vi "Main.vi"(10 "Sub Panel":refnum<vi>, 11 "Module Admin":refnum<class "Delacor_lib_QMH_Module Admin.lvclass">) -> ()   [LabVIEW 2020, in "Message Pane.lvlib"]
doc: "This template is based off of the Queued Message Handler design pattern and the Queued Message Handler project template that ships with LabVIEW.\n\nThe main difference is that the queue is private to this module and communication between modules is performed via Broadcast and Request events.\n\nRequest events are wrapped in public API methods and are handled in the Event Handling Loop (EHL) of this VI. Any module can register for Broadcast events sent by this module. The EHL generates messages based on user interface actions.\n\nThe Message Handling Loop (MHL) processes messages generated by the EHL, or by other messages. The messages are string values, so new messages can be added easily to the Message Cases case structure in the MHL. Each message cluster can also provide an optional value for Message Data, which is a variant that can be converted to whatever message-specific data is required.\n_____\nBased on Delacor QMH Project Template 5.0.0.82."
uses:
  Message Pane.lvlib
  <vilib>/Delacor/Delacor QMH/Libraries/Module Admin_class/Delacor_lib_QMH_Module Admin.lvclass
  Module Data--cluster.ctl
  Stop Argument--cluster.ctl
  <vilib>/Delacor/Delacor QMH/Libraries/Message Queue_class/Delacor_lib_QMH_Message Queue.lvclass/Delacor_lib_QMH_Message Queue.ctl
  <vilib>/Delacor/Delacor QMH/Libraries/Module Admin_class/Delacor_lib_QMH_Module Admin.lvclass/Delacor_lib_QMH_Module Admin.ctl
  Credit Update Argument--cluster.ctl
  Purchase action Argument--cluster.ctl
  SQLITE Inventory/Invetory Data Type.ctl
  <vilib>/Utility/miscctls.llb/LVPointTypeDef.ctl
  <vilib>/Delacor/Delacor QMH/Libraries/Message Queue_class/Delacor_lib_QMH_Enqueue Message (Single).vi
  <vilib>/Delacor/Delacor QMH/Libraries/Module Admin_class/Delacor_lib_QMH_Get External Launch.vi
  <vilib>/Utility/error.llb/Error Cluster From Error Code.vi
  <vilib>/ErrorRing/Error Ring.xnode
  <vilib>/Delacor/Delacor QMH/Libraries/Message Queue_class/Delacor_lib_QMH_Message Queue.lvclass
  SQLITE Inventory/SQLITE Inventory.lvlib
  Product Selecting Pane/Product Selecting Pane.lvlib
panel:
  out "Change":dbl
  out "Status":string
  out "Selected Product":string
  out "Credit":dbl
  out "error out":errorcluster
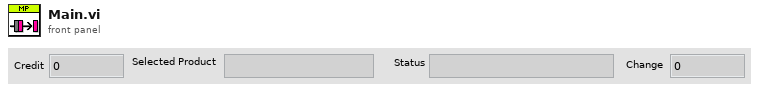
[diagram p1: front panel]
types:
  T1 = typedef "Message Pane.lvlib/Request Events--cluster.ctl" = cluster{"Stop Module":refnum<user-event>, "Show Panel":refnum<user-event>, "Hide Panel":refnum<user-event>, "Get Module Execution Status":refnum<user-event>, "Show Diagram":refnum<user-event>, "Credit Update":refnum<user-event>, "Purchase action":refnum<user-event>}
  T2 = typedef "Message Pane.lvlib/Module Data--cluster.ctl" = cluster{"Credit":dbl, "Status":string, "Change":dbl, "Product":string}
  T3 = enum32{"invalid lock state", "Not Locked", "Locked (No Password)", "Password-protected"}
  T4 = typedef "Message Pane.lvlib/Stop Argument--cluster.ctl" = cluster{"Origin":string, "Exit via Stop Module Req?":bool, "Wait for Module to stop?":bool}
  T5 = typedef "Message Pane.lvlib/Credit Update Argument--cluster.ctl" = cluster{"Numeric":dbl}
  T6 = typedef "Message Pane.lvlib/Purchase action Argument--cluster.ctl" = cluster{"Cluster":T7}
  T7 = typedef "Invetory Data Type.ctl" = cluster{"Name":string, "Price":dbl, "Stock":dbl}
  T8 = typedef "LVPointTypeDef.ctl" = cluster{"Horizontal":i16, "Vertical":i16}
  T9 = enum32{"Invalid", "Standard", "Closed", "Hidden", "Minimized", "Maximized"}
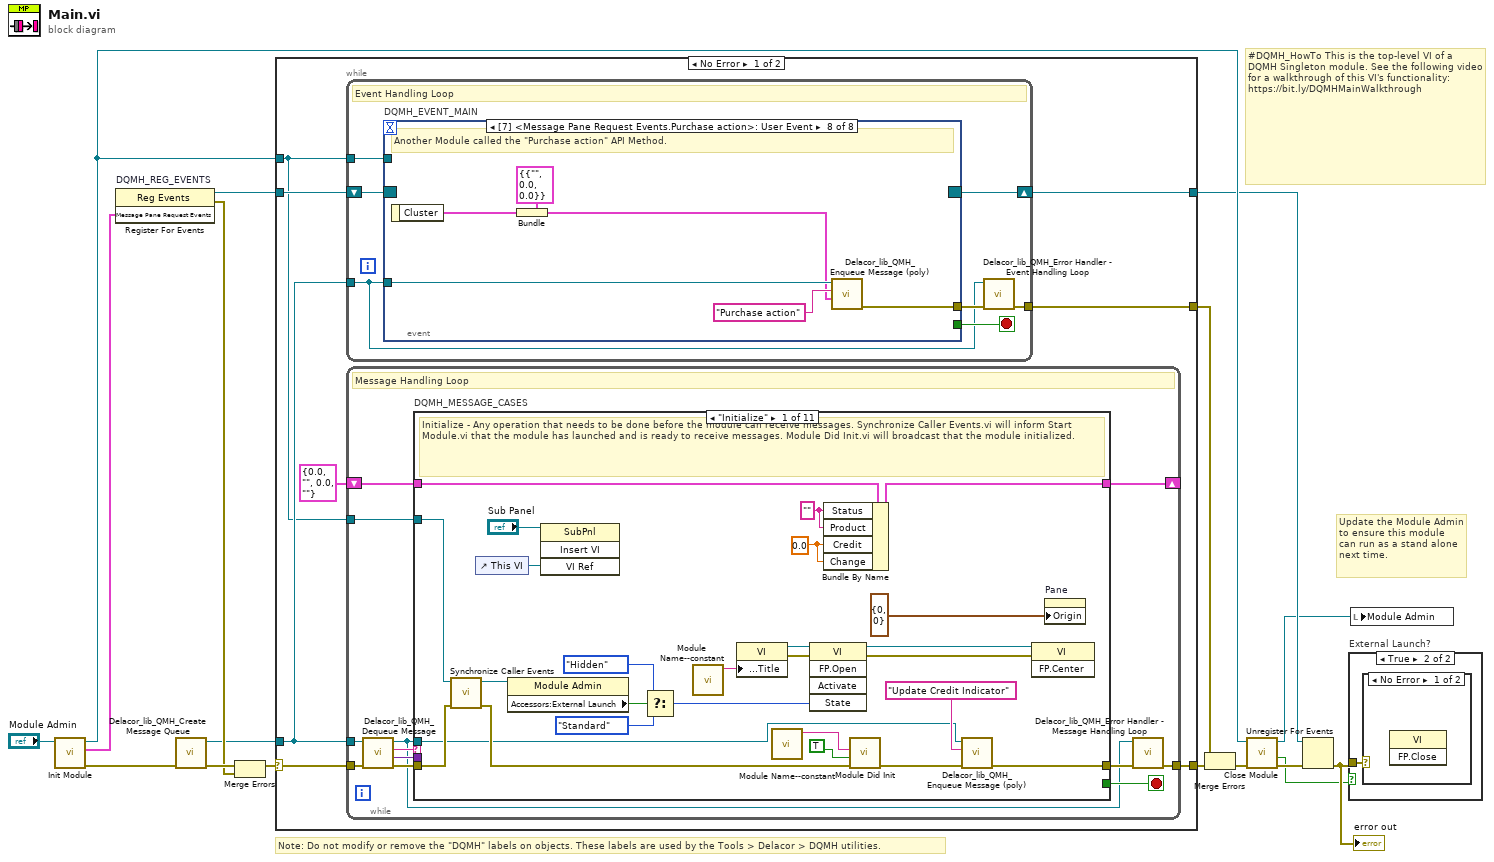
[diagram p0: block diagram]
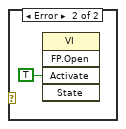
[diagram p3: hidden frame]
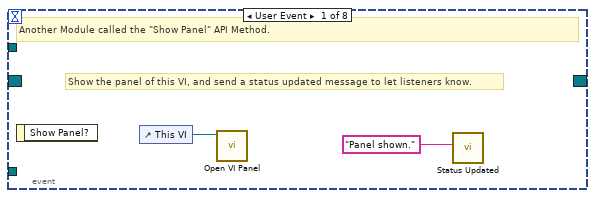
[diagram p4: hidden frame]
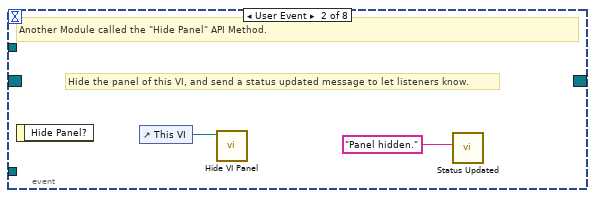
[diagram p5: hidden frame]
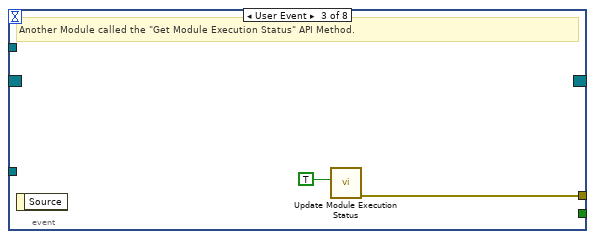
[diagram p6: hidden frame]
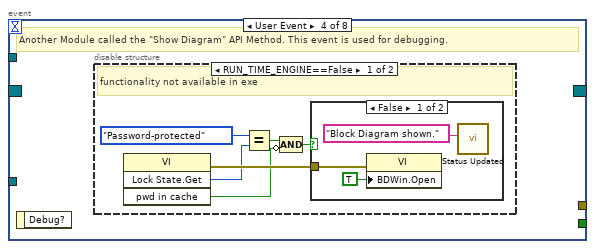
[diagram p7: hidden frame]
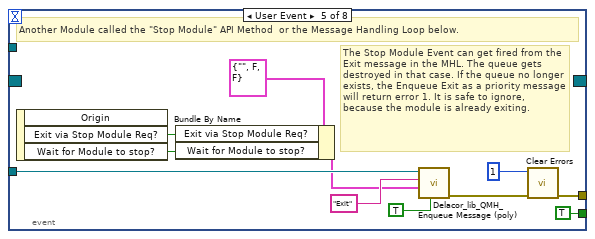
[diagram p10: hidden frame]
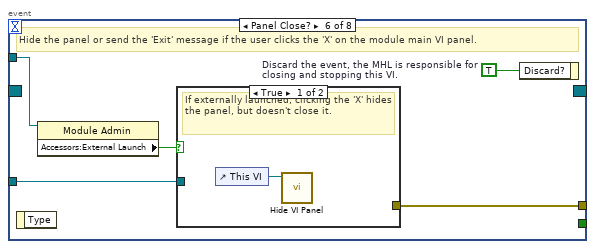
[diagram p11: hidden frame]
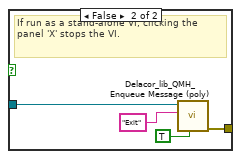
[diagram p12: hidden frame]
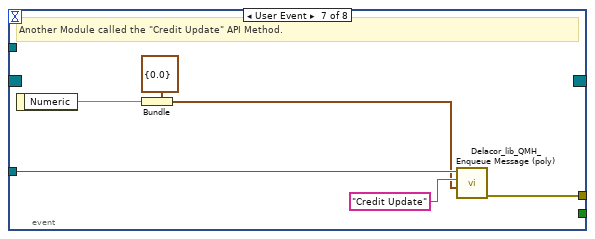
[diagram p13: hidden frame]
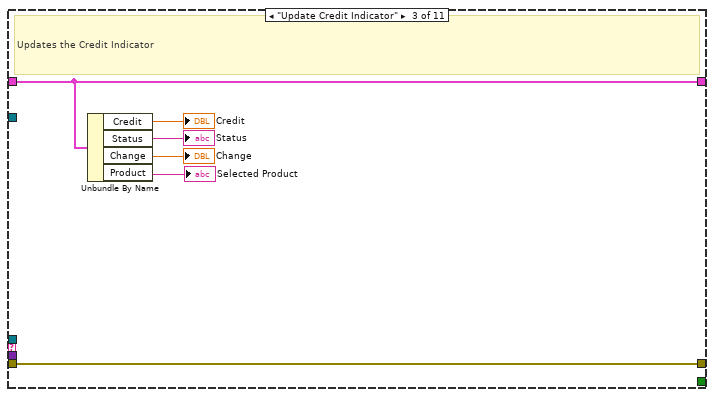
[diagram p15: hidden frame]
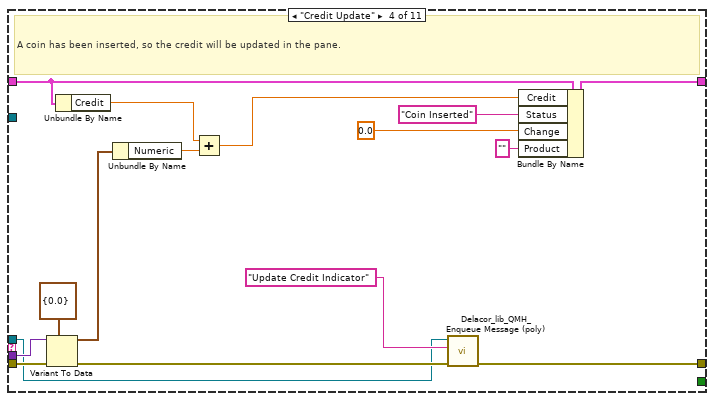
[diagram p16: hidden frame]
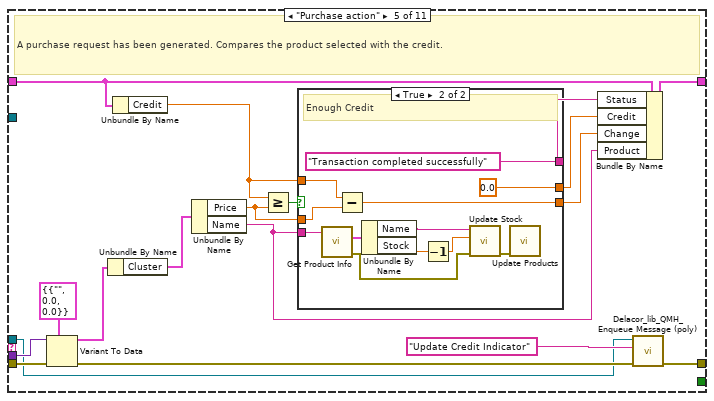
[diagram p17: hidden frame]
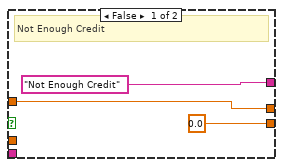
[diagram p18: hidden frame]
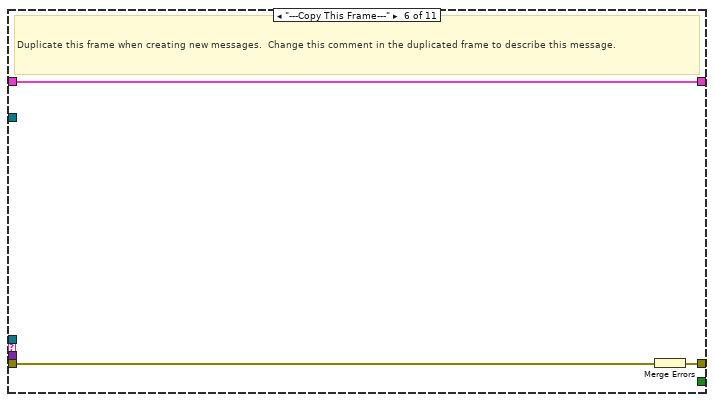
[diagram p19: hidden frame]
diagram:
  # "#DQMH_HowTo This is the top-level VI of a DQMH Singleton module. See the following video for a walkthrough of this VI's functionality: https://bit.ly/DQMHMainWalkthrough"
  # "Note: Do not modify or remove the \"DQMH\" labels on objects. These labels are used by the Tools > Delacor > DQMH utilities."
  # "Update the Module Admin to ensure this module can run as a stand alone next time."
  n1 = call "Init Module.vi"("Singleton Module Admin in"="Module Admin") -> ("error out"=w16:errorcluster, "Message Pane Request Events"=w5:T1, "Singleton Module Admin out"=w8:refnum<class "Delacor_lib_QMH_Module Admin.lvclass">)  [unwired: 8 in]
  n2 = register-events "DQMH_REG_EVENTS"(w5) -> (reference out=w6:refnum<event-registration>, error out=w9:errorcluster)  [unwired: 2 in]
  n3 = call <vilib>:"Delacor_lib_QMH_Create Message Queue.vi"("error in (no error)"=w16) -> ("error out"=w11:errorcluster, "Message Queue"=w4:refnum<class "Delacor_lib_QMH_Message Queue.lvclass">)  [unwired: 9 in]
  n4 = Merge Errors(w11, w9) -> (w10:errorcluster)
  n5 = case shown="No Error" w10 {
    selector: w10 -> [w23 w241]
    tunnel: [w25 w240] -> w17
    tunnel: [w22 w246] -> w7
    tunnel: w6 -> [w20 w246]
    tunnel: w4 -> [w19 w239]
    tunnel: [w24 _] -> w14
    tunnel: w8 -> [w18 w242]
    frame No Error {
      n6 = while {
        tunnel: w19 -> [w26]
        shift-right: [w29] -> w22
        shift-left: w20 -> [w30]
        tunnel: [w31] -> w24
        tunnel: w18 -> [w27]
        stop <- w28 stop-if-true
        # "Event Handling Loop"
        n7 = event "DQMH_EVENT_MAIN" shown="[7] <Message Pane Request Events.Purchase action>: User Event" {
          selector: w30 -> [_ _ _ _ _ _ _ _]
          dyn-events: [_ _ _ _ _ _ _ _] -> w29
          timeout: _ -> [_ _ _ _ _ _ _ _]
          tunnel: [_ _ _ _ TRUE ("Discard?") _ _ _] -> w28
          tunnel: w26 -> [_ _ _ _ w54 w61 w74 w80]
          tunnel: [_ _ w38 _ w57 w63 w69 w75] -> w32
          tunnel: w27 -> [_ _ _ _ _ w60 _ _]
          event User Event {
            # "Show the panel of this VI, and send a status updated message to let listeners know."
            # "Another Module called the \"Show Panel\" API Method."
            n8 = event-data() -> ()  [unwired: 1 in, 1 out]
            n9 = control-ref of="This VI"() -> (w34:refnum<vi>)
            n10 = call "Open VI Panel.vi"("VI"=w34) -> ()  [unwired: 10 in, 1 out]
            n11 = call "Status Updated.vi"("Status"="Panel shown." ("format string")) -> ()  [unwired: 10 in, 1 out]
          }
          event User Event {
            # "Hide the panel of this VI, and send a status updated message to let listeners know."
            # "Another Module called the \"Hide Panel\" API Method."
            n12 = event-data() -> ()  [unwired: 1 in, 1 out]
            n13 = control-ref of="This VI"() -> (w36:refnum<vi>)
            n14 = call "Hide VI Panel.vi"("VI"=w36) -> ()  [unwired: 10 in, 1 out]
            n15 = call "Status Updated.vi"("Status"="Panel hidden." ("format string")) -> ()  [unwired: 10 in, 1 out]
          }
          event User Event {
            # "Another Module called the \"Get Module Execution Status\" API Method."
            n16 = event-data() -> ()  [unwired: 1 in, 1 out]
            n17 = call "Update Module Execution Status.vi"("Running?"=TRUE) -> ("error out"=w38:errorcluster)  [unwired: 10 in]
          }
          event User Event {
            # "Another Module called the \"Show Diagram\" API Method. This event is used for debugging."
            n18 = event-data() -> ()  [unwired: 1 in, 1 out]
            n19 = disable-structure shown="RUN_TIME_ENGINE==False" {
              frame condition #0 (active) {
                # "functionality not available in exe"
                n20 = invoke class="VI" method="Lock State.Get"() -> (error out=w44:errorcluster, "Get Lock State"=w43:T3, "pwd in cache"=w40:bool)  [unwired: 4 in, 1 out]
                n21 = Equal?(x=T3."Password-protected", y=w43) -> (x = y?=w41:bool)
                n22 = Compound Arithmetic op=AND(w41, invert w40) -> (w39:bool)
                n23 = case shown="False" w39 {
                  tunnel: w44 -> [w47 _]
                  frame False {
                    n24 = property class="VI"(error in=w47, "BDWin.Open"=TRUE ("Block Diagram Window:Open")) -> ()  [unwired: 1 in, 2 out]
                    n25 = call "Status Updated.vi"("Status"="Block Diagram shown." ("format string")) -> ()  [unwired: 10 in, 1 out]
                  }
                  frame True {
                    # "Password-protected VI, and the password is not in the cache. Do not show the diagram."
                  }
                }
              }
              frame condition #1 {
              }
            }
          }
          event User Event {
            # "The Stop Module Event can get fired from the Exit message in the MHL. The queue gets destroyed in that case. If the queue no longer exists, the Enqueue Exit as a priority message will return error 1. It is safe to ignore, because the module is already exiting."
            # "Another Module called the \"Stop Module\" API Method  or the Message Handling Loop below."
            n26 = event-data() -> ("Exit via Stop Module Req?"=w50:bool, "Wait for Module to stop?"=w49:bool)  [unwired: 1 in, 1 out]
            n27 = Bundle By Name(cluster=T4 {"Origin"="", "Exit via Stop Module Req?"=FALSE, "Wait for Module to stop?"=FALSE} ("Stop Argument"), "Exit via Stop Module Req?"=w50, "Wait for Module to stop?"=w49) -> (w48:T4)
            n28 = call-poly <vilib>:"Delacor_lib_QMH_Enqueue Message (poly).vi"("Priority Message? (F)"=TRUE, "Message Data"=w48, "Message"="Exit", "Message Queue in"=w54) -> ("error out"=w58:errorcluster)  [unwired: 6 in, 1 out]
            n29 = call <vilib>:"Clear Errors.vi"("error in (no error)"=w58, "specific error code to clear (0: all)"=1) -> ("error out"=w57:errorcluster)  [unwired: 4 in, 1 out]
          }
          event Panel Close? {
            w62 = TRUE  # Discard the event, the MHL is responsible for closing and stopping this VI.
            # "Hide the panel or send the 'Exit' message if the user clicks the 'X' on the module main VI panel."
            n30 = event-data() -> ()  [unwired: 1 in, 1 out]
            n31 = property class="Module Admin"(reference=w60) -> ("Accessors:External Launch"=w59:bool)  [unwired: 1 in, 2 out]
            n32 = case shown="True" w59 {
              tunnel: w61 -> [_ w67]
              tunnel: [_ w68] -> w63
              frame True {
                # "If externally launched, clicking the 'X' hides the panel, but doesn't close it."
                n33 = control-ref of="This VI"() -> (w64:refnum<vi>)
                n34 = call "Hide VI Panel.vi"("VI"=w64) -> ()  [unwired: 10 in, 1 out]
              }
              frame False {
                # "If run as a stand-alone VI, clicking the panel 'X' stops the VI."
                n35 = call-poly <vilib>:"Delacor_lib_QMH_Enqueue Message (poly).vi"("Priority Message? (F)"=TRUE, "Message"="Exit", "Message Queue in"=w67) -> ("error out"=w68:errorcluster)  [unwired: 7 in, 1 out]
              }
            }
            n36 = event-data("Discard?"=w62) -> ()  [unwired: 1 in, 1 out]
          }
          event User Event {
            # "Another Module called the \"Credit Update\" API Method."
            n37 = event-data() -> ("Numeric"=w70:dbl)  [unwired: 1 in]
            n38 = Bundle(cluster=T5 {"Numeric"=0.0} ("Credit Update Argument"), "Numeric"=w70) -> (w71:T5)
            n39 = call-poly <vilib>:"Delacor_lib_QMH_Enqueue Message (poly).vi"("Message Data"=w71, "Message"="Credit Update", "Message Queue in"=w74) -> ("error out"=w69:errorcluster)  [unwired: 7 in, 1 out]
          }
          event User Event {
            # "Another Module called the \"Purchase action\" API Method."
            n40 = event-data() -> ("Cluster"=w76:T7)  [unwired: 1 in]
            n41 = Bundle(cluster=T6 {"Cluster"={"Name"="", "Price"=0.0, "Stock"=0.0}} ("Purchase action Argument"), "Cluster"=w76) -> (w77:T6)
            n42 = call-poly <vilib>:"Delacor_lib_QMH_Enqueue Message (poly).vi"("Message Data"=w77, "Message"="Purchase action", "Message Queue in"=w80) -> ("error out"=w75:errorcluster)  [unwired: 7 in, 1 out]
          }
        }
        n43 = call-dynamic "Delacor_lib_QMH_Error Handler - Event Handling Loop.vi"("error in (no error)"=w32, "Message Queue in"=w26) -> ("dup error in"=w31:errorcluster)  [unwired: 8 in, 1 out]
      }
      n44 = while {
        tunnel: w19 -> [w83]
        shift-right: [w87] -> _
        shift-left: T2 {"Credit"=0.0, "Status"="", "Change"=0.0, "Product"=""} ("Data Cluster") -> [w88]
        tunnel: w23 -> [w91]
        tunnel: [w89] -> w25
        tunnel: w18 -> [w81]
        stop <- w86 stop-if-true
        # "Message Handling Loop"
        n45 = call-dynamic "Delacor_lib_QMH_Dequeue Message.vi"("error in (no error)"=w91, "Message Queue in"=w83) -> ("error out"=w90:errorcluster, "Message Data"=w84:variant, "Message"=w85:string, "Message Queue out"=w82:refnum<class "Delacor_lib_QMH_Message Queue.lvclass">)  [unwired: 6 in]
        n46 = case "DQMH_MESSAGE_CASES" shown="\"Initialize\"" w85 {
          selector: w85 -> [_ _ _ _ _ _ _ _ _ _ w226]
          tunnel: w82 -> [w95 _ _ w130 w145 _ _ _ w196 w218 _]
          tunnel: w90 -> [w116 w120 w126 w142 w160 w178 w180 w185 w203 w224 w228]
          tunnel: [w97 w120 w126 w133 w146 w177 w180 w184 w199 w221 w229] -> w92
          tunnel: w88 -> [w106 w119 w125 w137 w156 w176 w179 w182 w198 w217 w227]
          tunnel: [w105 w119 w125 w138 w154 w176 w179 w182 w198 w217 w227] -> w87
          tunnel: [_ _ _ _ _ _ _ _ _ w216 _] -> w86
          tunnel: w84 -> [_ _ _ w141 w159 _ _ _ w197 w215 _]
          tunnel: w81 -> [w107 _ _ _ _ _ _ _ w195 w210 _]
          frame "Initialize" {
            w99 = 0.0
            w100 = "" ("Status")
            # "Initialize - Any operation that needs to be done before the module can receive messages. Synchronize Caller Events.vi will inform Start Module.vi that the module has launched and is ready to receive messages. Module Did Init.vi will broadcast that the module initialized."
            n47 = call "Synchronize Caller Events.vi"("error in (no error)"=w116, "Singleton Module Admin in"=w107) -> ("error out"=w115:errorcluster, "Singleton Module Admin out"=w102:refnum<class "Delacor_lib_QMH_Module Admin.lvclass">)  [unwired: 8 in]
            n48 = control-ref of="This VI"() -> (w93:refnum<vi>)
            n49 = property class="Module Admin"(reference=w102) -> ("Accessors:External Launch"=w111:bool)  [unwired: 1 in, 2 out]
            n50 = invoke class="SubPnl" method="Insert VI"(reference="Sub Panel", "VI Ref"=w93) -> ()  [unwired: 2 in, 4 out]
            n51 = Select(t=T9."Hidden" ("State"), s=w111, f=T9."Standard" ("State")) -> (s? t:f=w108:T9)
            n52 = call "Module Name--constant.vi"() -> ("Module Name"=w114:string)  [unwired: 11 in]
            n53 = property class="VI"("Front Panel.Title"=w114) -> (reference out=w113:refnum<vi>, error out=w118:errorcluster)  [unwired: 2 in]
            n54 = call "Module Name--constant.vi"() -> ("Module Name"=w103:string)  [unwired: 11 in]
            n55 = invoke class="VI" method="FP.Open"(reference=w113, error in=w118, "State"=w108) -> (reference out=w112:refnum<vi>, error out=w117:errorcluster)  [unwired: 2 in, 3 out]
            n56 = Bundle By Name(cluster=w106, "Status"=w100, "Product"=w100, "Credit"=w99, "Change"=w99) -> (w105:T2)
            n57 = call "Module Did Init.vi"("error in (no error)"=w115, "Initialized?"=TRUE, "Origin"=w103) -> ("error out"=w98:errorcluster)  [unwired: 8 in]
            n58 = call-poly <vilib>:"Delacor_lib_QMH_Enqueue Message (poly).vi"("error in (no error)"=w98, "Message"="Update Credit Indicator", "Message Queue in"=w95) -> ("error out"=w97:errorcluster)  [unwired: 7 in, 1 out]
            n59 = invoke class="VI" method="FP.Center"(reference=w112, error in=w117) -> ()  [unwired: 1 in, 3 out]
            n60 = property on="Pane" class="Pane"("Origin"=T8 {"Horizontal"=0, "Vertical"=0}) -> ()  [unwired: 2 in, 2 out]
          }
          frame "--- Module Specific ---" {
            # "Separator -- The following cases handle messages specific to this Module."
          }
          frame "Update Credit Indicator" {
            # "Updates the Credit Indicator"
            n61 = Unbundle By Name(w125) -> ("Credit"=→"Credit":dbl, "Status"=→"Status":string, "Change"=→"Change":dbl, "Product"=→"Selected Product":string)
          }
          frame "Credit Update" {
            # "A coin has been inserted, so the credit will be updated in the pane."
            n62 = Variant To Data(error in=w142, type=T5 {"Numeric"=0.0} ("Credit Update Argument"), Variant=w141) -> (data=w139:T5, error out=w132:errorcluster)
            n63 = Unbundle By Name(w137) -> ("Credit"=w136:dbl)
            n64 = Unbundle By Name(w139) -> ("Numeric"=w135:dbl)
            n65 = Add(x=w136, y=w135) -> (x+y=w134:dbl)
            n66 = call-poly <vilib>:"Delacor_lib_QMH_Enqueue Message (poly).vi"("error in (no error)"=w132, "Message"="Update Credit Indicator", "Message Queue in"=w130) -> ("error out"=w133:errorcluster)  [unwired: 7 in, 1 out]
            n67 = Bundle By Name(cluster=w137, "Credit"=w134, "Status"="Coin Inserted", "Change"=0.0, "Product"="") -> (w138:T2)
          }
          frame "Purchase action" {
            # "A purchase request has been generated. Compares the product selected with the credit."
            n68 = Variant To Data(error in=w160, type=T6 {"Cluster"={"Name"="", "Price"=0.0, "Stock"=0.0}} ("Purchase action Argument"), Variant=w159) -> (data=w157:T6, error out=w147:errorcluster)
            n69 = Unbundle By Name(w157) -> ("Cluster"=w144:T7)
            n70 = Unbundle By Name(w156) -> ("Credit"=w151:dbl)
            n71 = Unbundle By Name(w144) -> ("Price"=w150:dbl, "Name"=w143:string)
            n72 = Greater Or Equal?(x=w151, y=w150) -> (x >= y?=w155:bool)
            n73 = case shown="True" w155 {
              tunnel: ["Not Enough Credit" "Transaction completed successfully"] -> w153
              tunnel: [w162 0.0] -> w152
              tunnel: w151 -> [w162 w173]
              tunnel: w150 -> [_ w172]
              tunnel: [0.0 w171] -> w149
              tunnel: w143 -> [_ w170]
              frame False {
                # "Not Enough Credit"
              }
              frame True {
                # "Enough Credit"
                n74 = call "Get Product Info.vi"("Name"=w170) -> ("error out"=w164:errorcluster, "Product Info"=w169:T7)  [unwired: 8 in, 1 out]
                n75 = Subtract(x=w173, y=w172) -> (x-y=w171:dbl)
                n76 = Unbundle By Name(w169) -> ("Name"=w168:string, "Stock"=w167:dbl)
                n77 = Decrement(x=w167) -> (x-1=w166:dbl)
                n78 = call "Update Stock.vi"("error in (no error)"=w164, "Stock"=w166, "Name"=w168) -> ("error out"=w165:errorcluster)  [unwired: 8 in]
                n79 = call "Update Products.vi"("error in (no error)"=w165) -> ()  [unwired: 10 in, 1 out]
              }
            }
            n80 = Bundle By Name(cluster=w156, "Status"=w153, "Credit"=w152, "Change"=w149, "Product"=w143) -> (w154:T2)
            n81 = call-poly <vilib>:"Delacor_lib_QMH_Enqueue Message (poly).vi"("error in (no error)"=w147, "Message"="Update Credit Indicator", "Message Queue in"=w145) -> ("error out"=w146:errorcluster)  [unwired: 7 in, 1 out]
          }
          frame "---Copy This Frame---" {
            # "Duplicate this frame when creating new messages.  Change this comment in the duplicated frame to describe this message."
            n82 = Merge Errors(w178) -> (w177:errorcluster)
          }
          frame "--- Exit and Error Handling---" {
            # "Separator - The following cases handle errors and exit messages."
          }
          frame "Simulate MHL Error" {
            # "#DQMH_HowTo The 'Simulate MHL Error' button  illustrates how the MHL handles errors. This event is instructional in nature and can be removed."
            # "Simulate an error occurring at the MHL"
            n83 = call "Module Name--constant.vi"() -> ("Module Name"=w181:string)  [unwired: 11 in]
            n84 = xnode "Error Ring"("parameter 0"=w181) -> ("error out"=w183:errorcluster)
            n85 = Merge Errors(w185, w183) -> (w184:errorcluster)
          }
          frame "Error" {
            # "#CodeRecommended - If you ever change the name of this \"Error\" message, you'll need to update the name in the Check Loop Error.vi as well."
            # "#CodeRecommended - If the module is running in standalone mode (External Launch = FALSE), this code will pop up an error dialog and call the 'Exit' message if an error occurs. Add more fine-grained error handling here."
            # "Error - Check the error message data and respond accordingly. This message is sent by the \"Error Handler\" VIs at the end of each loop in this application."
            n86 = property class="Module Admin"(reference=w195) -> ("Accessors:External Launch"=w194:bool)  [unwired: 1 in, 2 out]
            n87 = Variant To Data(error in=w203, type=errorcluster {"status"=FALSE, "code"=0, "source"=""} ("error constant"), Variant=w197) -> (data=w204:errorcluster, error out=w201:errorcluster)
            n88 = call "Module Name--constant.vi"() -> ("Module Name"=w193:string)  [unwired: 11 in]
            n89 = call "Error Reported.vi"("Additional Information"=w193, "Error"=w204) -> ()  [unwired: 9 in, 1 out]
            n90 = case shown="False" w194 {
              tunnel: [w209 _] -> w200
              tunnel: w196 -> [w207 _]
              tunnel: w204 -> [w208 _]
              frame False {
                # "If the module is running standalone, then pop up an error dialog and call the \"Exit\" message."
                n91 = call <vilib>:"Simple Error Handler.vi"("error in (no error)"=w208) -> ()  [unwired: 4 in, 5 out]
                n92 = call-poly <vilib>:"Delacor_lib_QMH_Enqueue Message (poly).vi"("Priority Message? (F)"=TRUE, "Message"="Exit", "Message Queue in"=w207) -> ("error out"=w209:errorcluster)  [unwired: 7 in, 1 out]
              }
              frame True {
                # "If the module was launched externally, calling the Error Reported broadcast VI is the only action performed by the \"Error\" message. The module's caller can then process the error appropriately."
              }
            }
            n93 = Merge Errors(w201, w200) -> (w199:errorcluster)
            n94 = local write "error out"(w199) -> ()
          }
          frame "Exit" {
            w214 = 91  # 91: not all Exit messages will have an argument
            w216 = TRUE  # Stop the VI
            # "Release the message queue reference"
            # "#CodeNeeded - Add any required cleanup code here"
            # "Exit - Exit the application."
            n95 = Variant To Data(error in=w224, type=T4 {"Origin"="", "Exit via Stop Module Req?"=FALSE, "Wait for Module to stop?"=FALSE} ("Stop Argument"), Variant=w215) -> (data=w212:T4, error out=w220:errorcluster)
            n96 = call <vilib>:"Clear Errors.vi"("error in (no error)"=w220, "specific error code to clear (0: all)"=w214) -> ("error out"=w223:errorcluster)  [unwired: 4 in, 1 out]
            n97 = control-ref of="This VI"() -> (w211:refnum<vi>)
            n98 = call-dynamic "Delacor_lib_QMH_Release Message Queue.vi"("error in (no error)"=w223, "Message Queue"=w218) -> ("error out"=w222:errorcluster)  [unwired: 9 in]
            n99 = call "Handle Exit.vi"("Stop Argument"=w212, "Admin in"=w210, "VI reference"=w211) -> ("error out"=w219:errorcluster)  [unwired: 7 in, 1 out]
            n100 = Merge Errors(w222, w219) -> (w221:errorcluster)
          }
          frame Default {
            # "'Default' case only runs if there is a message that isn't defined in any of the other cases.  Output a programming error."
            n101 = call "Module Name--constant.vi"() -> ("Module Name"=w225:string)  [unwired: 11 in]
            n102 = xnode "Error Ring"("parameter 0"=w226, "parameter 1"=w225) -> ("error out"=w230:errorcluster)
            n103 = Merge Errors(w228, w230) -> (w229:errorcluster)
          }
        }
        n104 = call-dynamic "Delacor_lib_QMH_Error Handler - Message Handling Loop.vi"("error in (no error)"=w92, "Message Queue in"=w82) -> ("dup error in"=w89:errorcluster)  [unwired: 8 in, 1 out]
      }
    }
    frame Error {
      # "Synchronize Caller Events.vi will inform Start Module.vi that the module has launched and will let the code calling Start Module.vi register for broadcasts and would permit the caller receive the broadcast that an error occurred at launch time."
      n105 = call-dynamic "Delacor_lib_QMH_Release Message Queue.vi"("error in (no error)"=w241, "Message Queue"=w239) -> ("error out"=w240:errorcluster)  [unwired: 9 in]
      n106 = call "Synchronize Caller Events.vi"("Singleton Module Admin in"=w242) -> ("error out"=w247:errorcluster)  [unwired: 9 in, 1 out]
      n107 = call "Module Name--constant.vi"() -> ("Module Name"=w245:string)  [unwired: 11 in]
      n108 = Format Into String(format string="An error occurred during initialization. %s is no longer running.", w245) -> (resulting string=w243:string)  [unwired: 2 in, 1 out]
      n109 = Merge Errors(w240, w247) -> (w248:errorcluster)
      n110 = call "Error Reported.vi"("Additional Information"=w243, "Error"=w248) -> ()  [unwired: 9 in, 1 out]
    }
  }
  n111 = Merge Errors(w14, w17) -> (w13:errorcluster)
  n112 = call "Close Module.vi"("error in (no error)"=w13, "Module Admin in"=w8) -> ("error out"=w15:errorcluster, "External Launch"=w1:bool, "Module Admin out"=w2:refnum<class "Delacor_lib_QMH_Module Admin.lvclass">)  [unwired: 7 in]
  n113 = Unregister For Events(event registration refnum=w7, error in=w15) -> (error out=w12:errorcluster)
  "error out" <- w12
  n114 = case "External Launch?" shown="True" w1 {
    tunnel: w12 -> [_ w249]
    frame False {
    }
    frame True {
      n115 = case shown="No Error" w249 {
        frame No Error {
          n116 = invoke class="VI" method="FP.Close"() -> ()  [unwired: 3 in, 3 out]
        }
        frame Error {
          n117 = invoke class="VI" method="FP.Open"("Activate"=TRUE ("Activate?")) -> ()  [unwired: 4 in, 5 out]
        }
      }
    }
  }
  n118 = local write "Module Admin"(w2) -> ()
